vi "macro_DigSeqLogic_Off_Delay.vi"   [LabVIEW 2019, in "Trajectory_Library.lvlib"]
uses:
  Trajectory_Library.lvlib
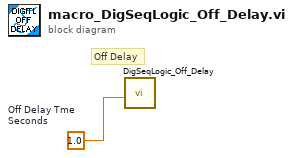
[diagram p0: block diagram]
diagram:
  w1 = 1.0  # Off Delay Tme Seconds
  # "Off Delay"
  n1 = call "DigSeqLogic_Off_Delay.vi"("Delay"=w1) -> ()  [unwired: 9 in, 2 out]
